vi "Configure Operational Mode.vi"(8 "error in (no error)":errorcluster, 9 "Operational Mode":u8(ring) items=["Enter Run Mode (from Standby Mode)"=117, "Enter Standby Mode (from Run Mode)"=118, "Enter Sleep Mode (from Run Mode)"=131, "Exit Sleep Mode"=132], 11 "Honeywell Compass HMC6343":refnum<class "Honeywell Compass HMC6343.lvclass">) -> (0 "error out":errorcluster, 3 "Honeywell Compass HMC6343 out":refnum<class "Honeywell Compass HMC6343.lvclass">)   [LabVIEW 2019, in "Honeywell Compass HMC6343.lvclass"]
doc: "Changes the Operational Mode of the device. There are three Operational Modes : Run Mode, Standby Mode and Sleep Mode. Sleep mode is defined as having the analog circuitry powered off, and has the lowest power consumption while power is applied to the VDD pins. Standby mode has the HMC6343 fully powered, but with no measurements performed and the processor is waiting for commands to perform. Run mode is fully engaged in continuous measurements at the set rate, and ready to receive further commands."
uses:
  Honeywell Compass HMC6343.lvclass
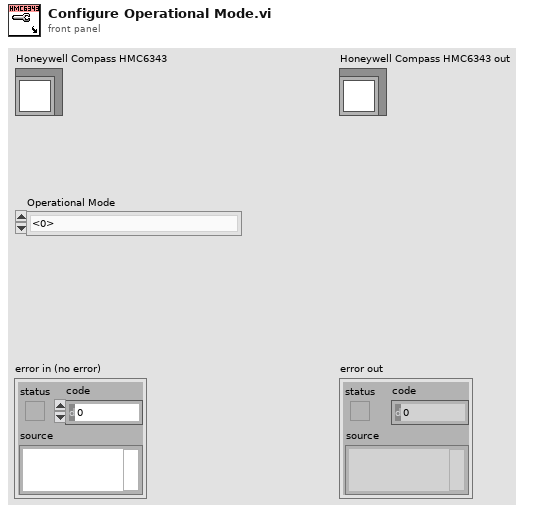
[diagram p1: front panel]
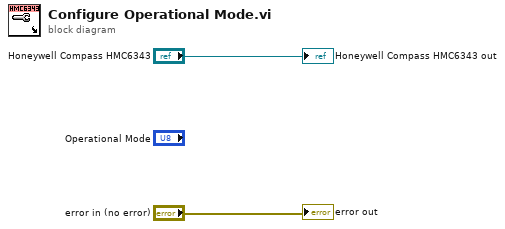
[diagram p0: block diagram]
diagram:
  "error out" <- "error in (no error)"
  "Honeywell Compass HMC6343 out" <- "Honeywell Compass HMC6343"
